vi "Get Result.vi"(8 "error in (no error)":errorcluster, 11 "Pulse Recorder in":refnum<class "Pulse Recorder.lvclass">) -> (0 "error out":errorcluster, 2 "Data Result":refnum<class "Acquired Result.lvclass">, 3 "Pulse Recorder out":refnum<class "Pulse Recorder.lvclass">)   [LabVIEW 2015]
uses:
  NHMFL_Core/Libraries/Instruments/Pulse Driver/Pulse Driver.lvclass
  Results/Acquired Result/Acquired Result.lvclass
  Pulse Recorder.lvclass
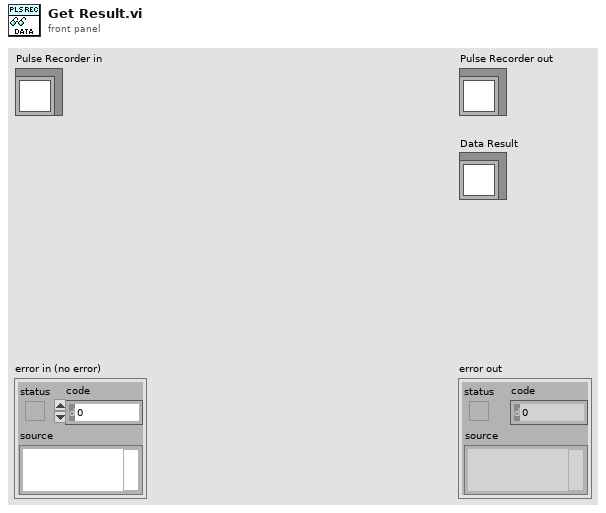
[diagram p1: front panel]
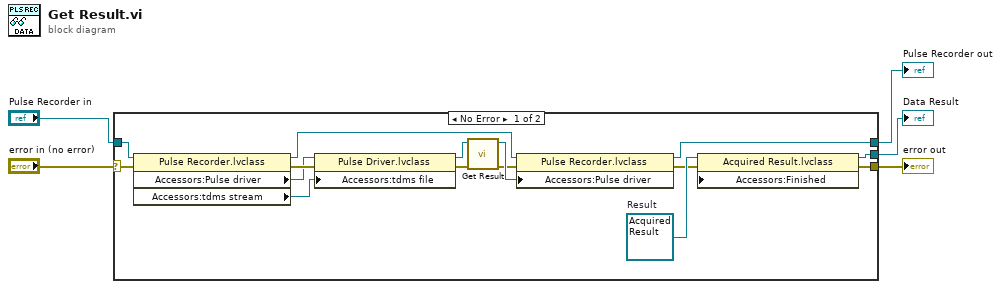
[diagram p0: block diagram]
diagram:
  n1 = case shown="No Error" "error in (no error)" {
    selector: "error in (no error)" -> [w12 w22]
    tunnel: [w7 w22] -> w4
    tunnel: [w10 w21] -> w2
    tunnel: "Pulse Recorder in" -> [w11 w21]
    tunnel: [w6 _] -> w1
    frame No Error {
      w9 = refnum<class "Acquired Result.lvclass"> refnum  # Result
      n2 = property class="Pulse Recorder.lvclass"(reference=w11, error in=w12) -> (reference out=w20:refnum<class "Pulse Recorder.lvclass">, error out=w19:errorcluster, "Accessors:Pulse driver"=w18:refnum<class "Pulse Driver.lvclass">, "Accessors:tdms stream"=w17:refnum<k34>)
      n3 = property class="Pulse Driver.lvclass"(reference=w18, error in=w19, "Accessors:tdms file"=w17) -> (reference out=w16:refnum<class "Pulse Driver.lvclass">, error out=w14:errorcluster)
      n4 = call-dynamic "Get Result.vi"("error in (no error)"=w14, "Pulse Driver in"=w16) -> ("error out"=w13:errorcluster, "Pulse Driver out"=w15:refnum<class "Pulse Driver.lvclass">)  [unwired: 7 in, 1 out]
      n5 = property class="Pulse Recorder.lvclass"(reference=w20, error in=w13, "Accessors:Pulse driver"=w15) -> (reference out=w10:refnum<class "Pulse Recorder.lvclass">, error out=w8:errorcluster)
      n6 = property class="Acquired Result.lvclass" props=["Accessors:Finished"](reference=w9, error in=w8) -> (reference out=w6:refnum<class "Acquired Result.lvclass">, error out=w7:errorcluster)  [unwired: 1 in]
    }
    frame Error {
    }
  }
  "error out" <- w4
  "Pulse Recorder out" <- w2
  "Data Result" <- w1
